vi "Instantiate Py Doc.vi"(5 "Py File Path":path, 11 "error in (no error)":errorcluster) -> (4 "Py Editor.lvclass":refnum<class "Py Editor.lvclass">, 6 "Py Shell.lvclass":refnum<class "Py Shell.lvclass">, 15 "error out":errorcluster)   [LabVIEW 2016, in "Py Doc.lvclass"]
uses:
  Py Doc.lvclass
  Child Classes/Py Editor/Py Editor.lvclass
  Child Classes/Py Shell/Py Shell.lvclass
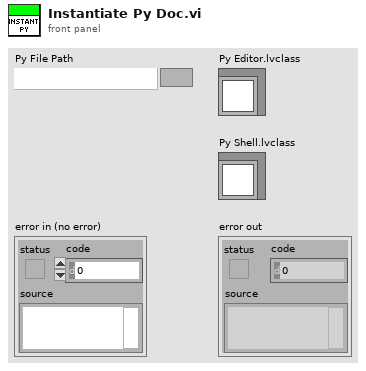
[diagram p1: front panel]
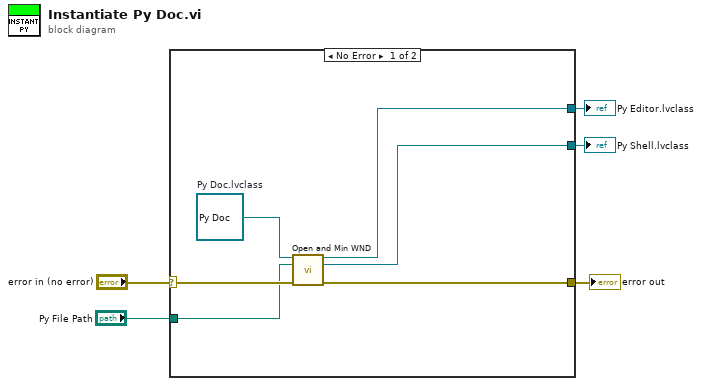
[diagram p0: block diagram]
diagram:
  n1 = case shown="No Error" "error in (no error)" {
    selector: "error in (no error)" -> [w8 w12]
    tunnel: [w11 w12] -> w4
    tunnel: "Py File Path" -> [w6 _]
    tunnel: [w10 _] -> w2
    tunnel: [w9 _] -> w1
    frame No Error {
      w7 = refnum<class "Py Doc.lvclass"> refnum  # Py Doc.lvclass
      n2 = call "Open and Min WND.vi"("Py Doc in"=w7, "Document Path"=w6, "error in (no error)"=w8) -> ("Py Editor.lvclass"=w10:refnum<class "Py Editor.lvclass">, "Py Shell.lvclass"=w9:refnum<class "Py Shell.lvclass">, "error out"=w11:errorcluster)  [unwired: 10 in]
    }
    frame Error {
    }
  }
  "error out" <- w4
  "Py Editor.lvclass" <- w2
  "Py Shell.lvclass" <- w1
